vi "IPI_CalLaserValue.vi"(8 "index":dbl, 9 "CurrentValue":string, 10 "LaserBase":string, 11 "Laserarray":string[](array[string])) -> (3 "Laservalue_result":string)   [LabVIEW 2015]
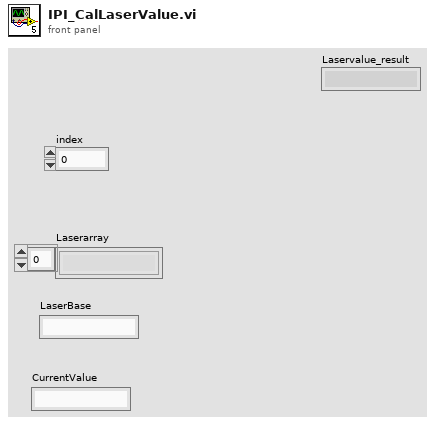
[diagram p1: front panel]
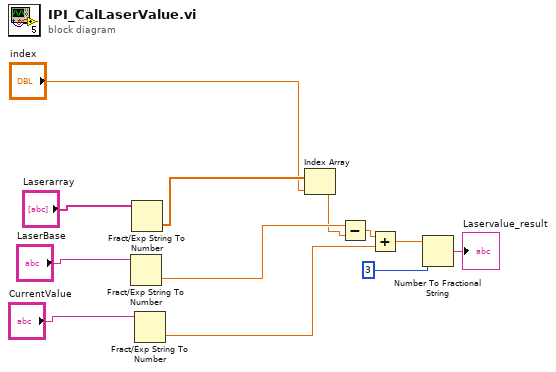
[diagram p0: block diagram]
diagram:
  n1 = Fract/Exp String To Number(string="LaserBase") -> (number=w5:dbl)  [unwired: 3 in, 1 out]
  n2 = Fract/Exp String To Number(string="Laserarray") -> (number=w9:dbl[])  [unwired: 3 in, 1 out]
  n3 = Fract/Exp String To Number(string="CurrentValue") -> (number=w2:dbl)  [unwired: 3 in, 1 out]
  n4 = Index Array(array=w9, index="index") -> (element=w4:dbl)
  n5 = Subtract(x=w5, y=w4) -> (x-y=w3:dbl)
  n6 = Add(x=w3, y=w2) -> (x+y=w1:dbl)
  n7 = Number To Fractional String(number=w1, precision (6)=i16 3 ("精度(6)")) -> (F-format string=→"Laservalue_result":string)  [unwired: 2 in]
